vi "Write 7z.bat.vi"(8 "error in (no error)":errorcluster, 11 "PostBuildSupport in":refnum<class "PostBuildSupport.lvclass">) -> (0 "error out":errorcluster, 3 "PostBuildSupport out":refnum<class "PostBuildSupport.lvclass">)   [LabVIEW 2016, in "PostBuildSupport.lvclass"]
uses:
  PostBuildSupport.lvclass
  PostBuildSupport.lvclass/PostBuildSupport.ctl
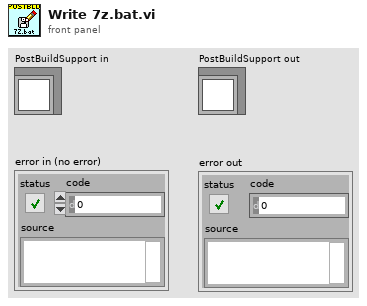
[diagram p1: front panel]
types:
  T1 = enum16{"open", "replace", "create", "open or create", "replace or create", "replace or create with confirmation"}
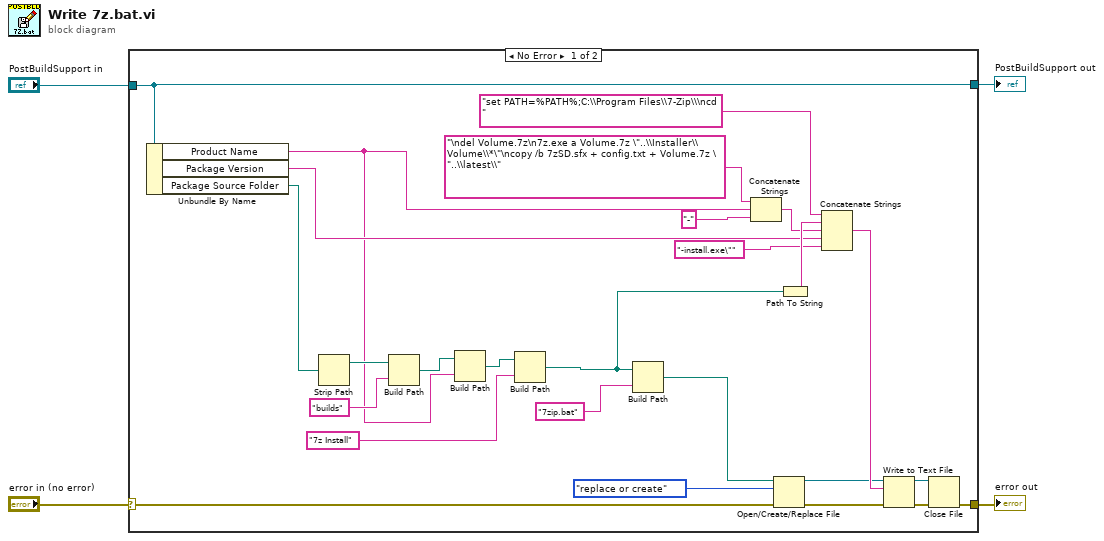
[diagram p0: block diagram]
diagram:
  n1 = case shown="No Error" "error in (no error)" {
    selector: "error in (no error)" -> [w6 w32]
    tunnel: [w20 w32] -> w4
    tunnel: "PostBuildSupport in" -> [w5 w31]
    tunnel: [w5 w31] -> w1
    frame No Error {
      n2 = Unbundle By Name(w5) -> ("Product Name"=w10:string, "Package Version"=w14:string, "Package Source Folder"=w13:path)
      n3 = Strip Path(path=w13) -> (stripped path=w27:path)  [unwired: 1 out]
      n4 = Build Path(base path=w27, name or relative path="builds") -> (appended path=w11:path)
      n5 = Build Path(base path=w11, name or relative path=w10) -> (appended path=w9:path)
      n6 = Build Path(base path=w9, name or relative path="7z Install") -> (appended path=w7:path)
      n7 = Build Path(base path=w7, name or relative path="7zip.bat") -> (appended path=w25:path)
      n8 = Concatenate Strings("\ndel Volume.7z\n7z.exe a Volume.7z \"..\\Installer\\Volume\\*\"\ncopy /b 7zSD.sfx + config.txt + Volume.7z \"..\\latest\\" ("Name of target (My Computer)"), w10, "-" ("Name of target (My Computer)")) -> (w16:string)
      n9 = Open/Create/Replace File(file path (use dialog)=w25, error in=w6, operation (0:open)=T1."replace or create") -> (refnum out=w26:refnum<file>, error out=w24:errorcluster)  [unwired: 3 in, 1 out]
      n10 = Path To String(path=w7) -> (string=w19:string)
      n11 = Concatenate Strings("set PATH=%PATH%;C:\\Program Files\\7-Zip\\\ncd " ("Name of target (My Computer)"), w19, w16, w14, "-install.exe\"" ("Name of target (My Computer)")) -> (w30:string)
      n12 = Write to Text File(file (use dialog)=w26, text=w30, error in=w24) -> (refnum out=w21:refnum<file>, error out=w22:errorcluster)  [unwired: 1 in, 1 out]
      n13 = Close File(refnum=w21, error in=w22) -> (error out=w20:errorcluster)  [unwired: 1 out]
    }
    frame Error {
    }
  }
  "error out" <- w4
  "PostBuildSupport out" <- w1
